vi "Abort.vi"(8 "error in (no error)":errorcluster, 11 "Execution API In":refnum<class "Execution API.lvclass">) -> (0 "error out":errorcluster, 3 "Execution API Out":refnum<class "Execution API.lvclass">)   [LabVIEW 2020, in "Execution API.lvclass"]
doc: "Aborts a running execution."
uses:
  Execution API.lvclass
  Execution API.lvclass/Execution API.ctl
  Test Runner/Test Runner.lvclass
  Plugin/Plugin.lvclass
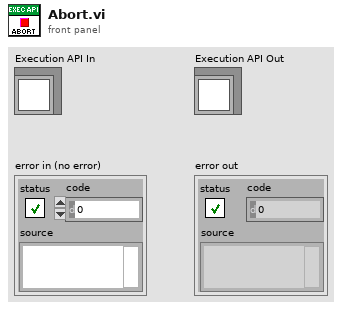
[diagram p1: front panel]
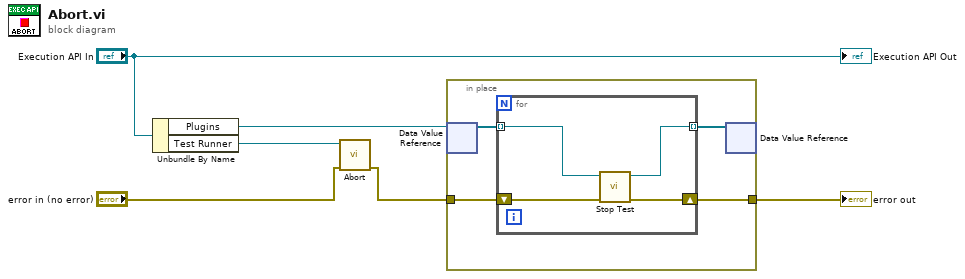
[diagram p0: block diagram]
diagram:
  n1 = Unbundle By Name("Execution API In") -> ("Plugins"=w1:refnum<data-value>, "Test Runner"=w3:refnum<class "Test Runner.lvclass">)
  n2 = call-dynamic "Abort.vi"("error in (no error)"="error in (no error)", "Test Runner in"=w3) -> ("error out"=w6:errorcluster)  [unwired: 9 in]
  n3 = in-place {
    in-place-border: w6 -> [w10]
    in-place-border: [w9] -> w4
    n4 = in-place-dvr #1(w1) -> (w8:refnum<class "Plugin.lvclass">[])  [unwired: 1 out]
    n5 = for {
      shift-right: [w13] -> w9
      shift-left: w10 -> [w14]
      tunnel: [w12] -> w7 mode=indexing
      tunnel: w8 -> [w11] mode=indexing
      n6 = call-dynamic "Stop Test.vi"("error in (no error)"=w14, "Plugin in"=w11) -> ("error out"=w13:errorcluster, "Plugin out"=w12:refnum<class "Plugin.lvclass">)  [unwired: 8 in]
    }
    n7 = in-place-dvr #1(w7) -> ()  [unwired: 2 out]
  }
  "error out" <- w4
  "Execution API Out" <- "Execution API In"
